vi "exnSharedSub string to floating point variant.vi"(0 "type as string":string, 7 "Variant in":variant) -> (8 "Variant out":variant)   [LabVIEW 2017]
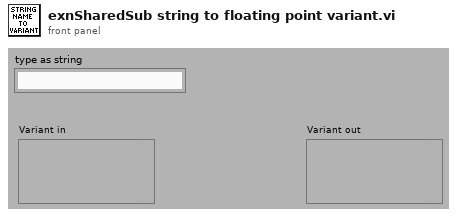
[diagram p1: front panel]
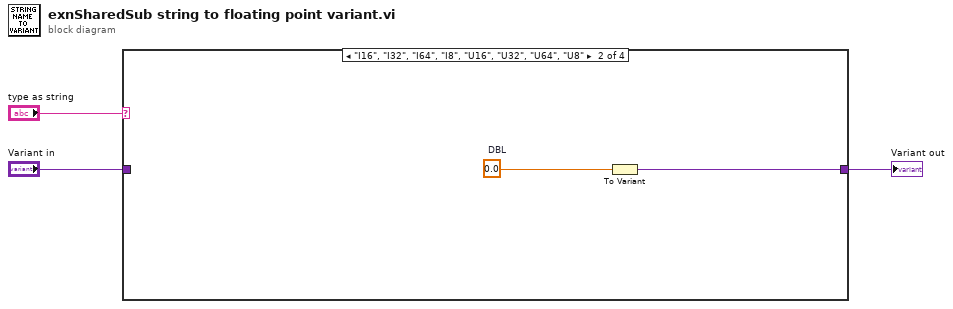
[diagram p0: block diagram]
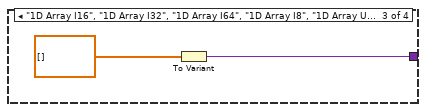
[diagram p3: hidden frame]
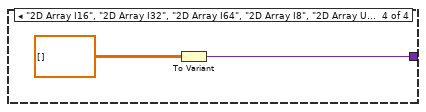
[diagram p4: hidden frame]
diagram:
  n1 = case shown="\"I16\", \"I32\", \"I64\", \"I8\", \"U16\", \"U32\", \"U64\", \"U8\"" "type as string" {
    tunnel: [w4 w5 w8 w10] -> w2
    tunnel: "Variant in" -> [w4 _ _ _]
    frame Default {
      # "Result type is already floating point"
    }
    frame "I16", "I32", "I64", "I8", "U16", "U32", "U64", "U8" {
      w6 = 0.0  # DBL
      n2 = To Variant(anything=w6) -> (Variant=w5:variant)
    }
    frame "1D Array I16", "1D Array I32", "1D Array I64", "1D Array I8", "1D Array U16", "1D Array U32", "1D Array U64", "1D Array U8" {
      n3 = To Variant(anything=dbl[] []) -> (Variant=w8:variant)
    }
    frame "2D Array I16", "2D Array I32", "2D Array I64", "2D Array I8", "2D Array U16", "2D Array U32", "2D Array U64", "2D Array U8" {
      n4 = To Variant(anything=dbl[][] []) -> (Variant=w10:variant)
    }
  }
  "Variant out" <- w2
